vi "Inspect Call.vi"(7 "Actor in":refnum<data-value>, 9 "Teller":T1 {"Absolute Time" format="%<%x %.3X>T"}, 10 "Msg":refnum<class "Msg.lvclass">) -> (0 "Error out":errorcluster, 5 "Actor out":refnum<data-value>)   [LabVIEW 2020, in "jettl.lvlib"]
uses:
  jettl.lvlib
  Actor/Actor.lvclass
  Msg/Msg.lvclass
  Msg Set.ctl
  Refs/Refs.lvclass
  Actor.ctl
  Unified Actor Relation.ctl
  Teller.ctl
  Msgs.ctl
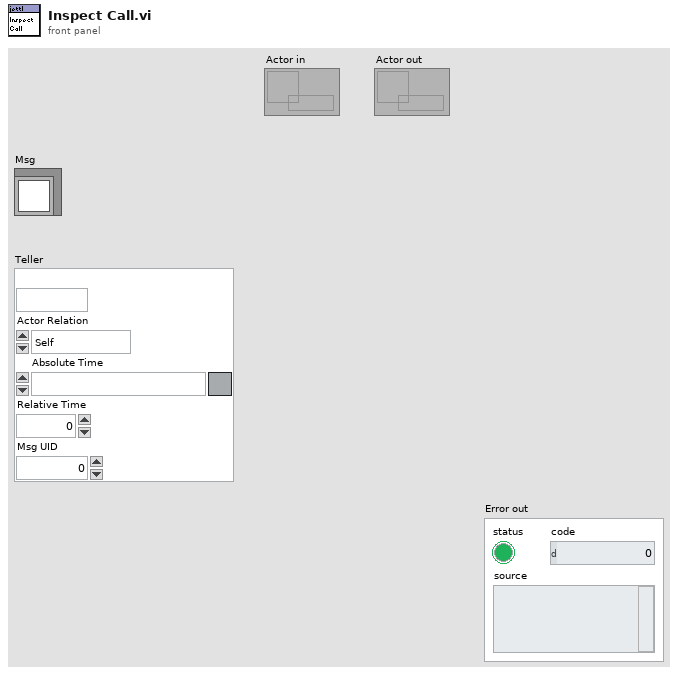
[diagram p1: front panel]
types:
  T1 = typedef "jettl.lvlib/Teller.ctl" = cluster{"Unified Actor Alias":string, "Actor Relation":T2, "Absolute Time":timestamp, "Relative Time":dbl, "Msg UID":i32}
  T2 = typedef "jettl.lvlib/Unified Actor Relation.ctl" = enum16{"Self", "Parent", "Child"}
  T3 = typedef "jettl.lvlib/Actor.ctl" = cluster{"Msgs":T4, "Leaf":bool, "Index":i32, "Actor":refnum<class "Actor.lvclass">, "Refs":refnum<class "Refs.lvclass">}
  T4 = typedef "jettl.lvlib/Msgs.ctl" = cluster{"Inbound":T5, "Outbound":T5, "Implemented":T5, "Tell Init":T5, "Tell Init Self":T5, "Tell Init Parent":T5, "Tell Init Child":T5, "Tell Forward":T5, "Tell Forward Self":T5, "Tell Forward Parent":T5, "Tell Forward Child":T5}
  T5 = typedef "jettl.lvlib/Msg Set.ctl" = set{refnum<class "Msg.lvclass">}
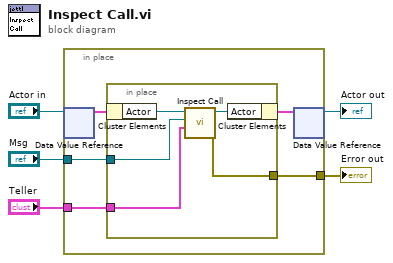
[diagram p0: block diagram]
diagram:
  n1 = in-place {
    in-place-border: [w8] -> w3
    in-place-border: "Teller" -> [w7]
    in-place-border: "Msg" -> [w6]
    n2 = in-place-dvr #1("Actor in") -> (w10:T3)  [unwired: 1 out]
    n3 = in-place {
      in-place-border: [w13] -> w8
      in-place-border: w7 -> [w12]
      in-place-border: w6 -> [w11]
      n4 = in-place-cluster #2(w10) -> ("Actor"=w15:refnum<class "Actor.lvclass">)
      n5 = call-dynamic "Inspect Call.vi"("Teller"=w12, "Msg"=w11, "Actor in"=w15) -> ("Error out"=w13:errorcluster, "Actor out"=w14:refnum<class "Actor.lvclass">)  [unwired: 7 in]
      n6 = in-place-cluster #2("Actor"=w14) -> (w9:T3)
    }
    n7 = in-place-dvr #1(w9) -> (→"Actor out":refnum<data-value>)  [unwired: 1 out]
  }
  "Error out" <- w3
